vi "calc_inner.vi"(11 "Qube":refnum<class "System.lvclass">) -> (3 "Qube":refnum<class "System.lvclass">)   [LabVIEW 2021, in "System.lvclass"]
uses:
  System.lvclass
  System.lvclass/System.ctl
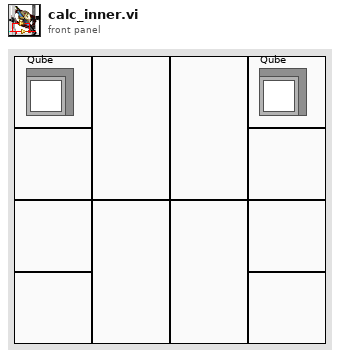
[diagram p1: front panel]
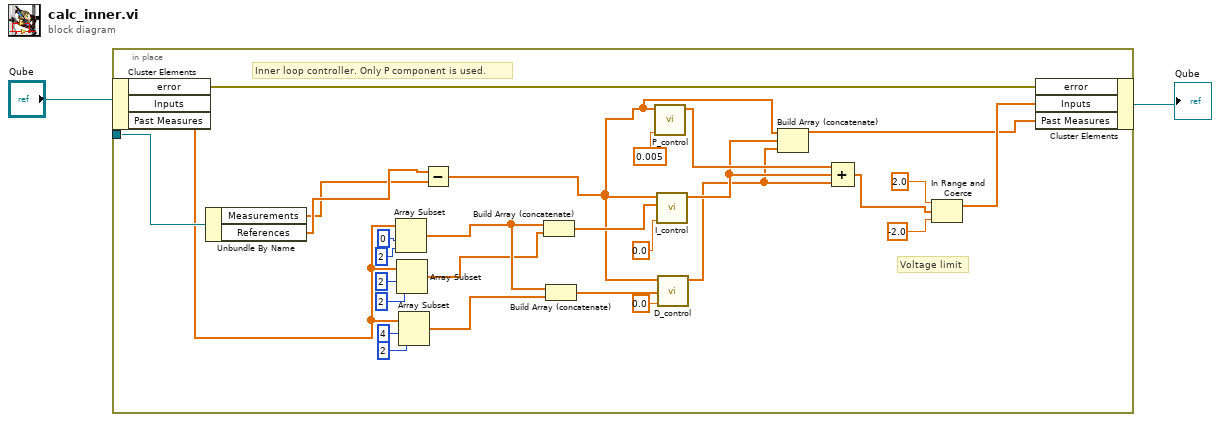
[diagram p0: block diagram]
diagram:
  n1 = in-place {
    in-place-border: "Qube" -> [w29]
    # "Inner loop controller. Only P component is used."
    # "Voltage limit"
    n2 = in-place-cluster #1("Qube") -> ("error"=w30:errorcluster, "Past Measures"=w22:dbl[])  [unwired: 1 out]
    n3 = Unbundle By Name(w29) -> ("Measurements"=w27:dbl[], "References"=w28:dbl[])
    n4 = Array Subset(array=w22, index=0, length=2) -> (w15:dbl[])
    n5 = Array Subset(array=w22, index=2, length=2) -> (w14:dbl[])
    n6 = Array Subset(array=w22, index=4, length=2) -> (w13:dbl[])
    n7 = Subtract(x=w28, y=w27) -> (x-y=w6:dbl[])
    n8 = Build Array (concatenate)(w15, w14) -> (w20:dbl[])
    n9 = Build Array (concatenate)(w15, w13) -> (w16:dbl[])
    n10 = call "P_control.vi"("Kp"=0.005, "Feedback error"=w6) -> ("P control"=w18:dbl[])  [unwired: 9 in]
    n11 = call "I_control.vi"("Ki"=0.0, "Past measures"=w20, "Feedback error"=w6) -> ("I control"=w5:dbl[])  [unwired: 8 in]
    n12 = call "D_control.vi"("Kd"=0.0, "Past Measures"=w16, "Feedback error"=w6) -> ("D control"=w4:dbl[])  [unwired: 8 in]
    n13 = Build Array (concatenate)(w6, w5, w4) -> (w3:dbl[])
    n14 = Compound Arithmetic op=ADD(w18, w5, w4) -> (w26:dbl[])
    n15 = In Range and Coerce(upper limit=2.0, x=w26, lower limit=-2.0) -> (coerced(x)=w23:dbl[])  [unwired: 1 out]
    n16 = in-place-cluster #1("error"=w30, "Inputs"=w23, "Past Measures"=w3) -> (→"Qube":refnum<class "System.lvclass">)
  }
